vi "SUB_NI_Close_COM9.vi"() -> (0 "error":i32)   [LabVIEW 2011]
doc: "Closes the specified port."
panel:
  # "Problem: \nI want to make LabVIEW temporarily give up access to a serial port so that other programs can access it, \nbut I can't find a VI that will close my serial port. How can I do this?\n\nSolution: \nYou can use a lower level serial VI called Close Serial Driver.vi. \nIn LabVIEW 5.x, this VI is found under \\Labview\\vi.lib\\Instr\\_sersup.llb. In LabVIEW 6.0, \nit is located under \\LabVIEW 6\\vi.lib\\instr\\Serial.llb. If you include this VI in the application, \nit will allow other programs to use the serial port without having to exit LabVIEW. You can then re-access the port in LabVIEW by \nsubsequently running Serial Port Init.vi, and Serial Write.vi, or Serial Read.vi. \n\nOpening and closing serial ports in LabVIEW can also be done using VISA. This is done with VISA Open.vi and VISA Close.vi."
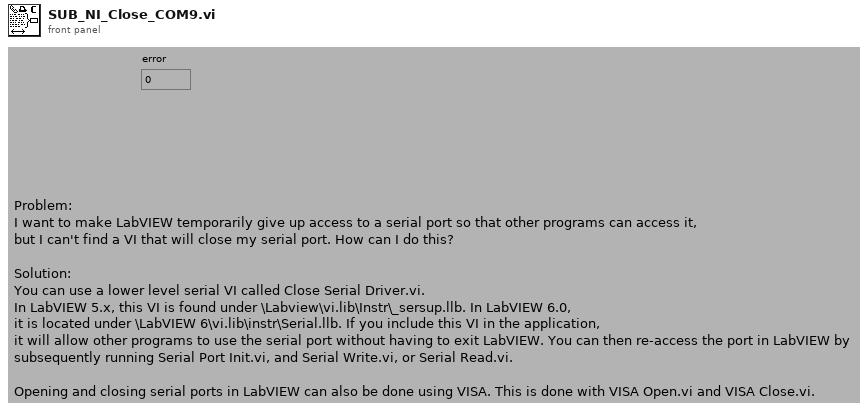
[diagram p1: front panel]
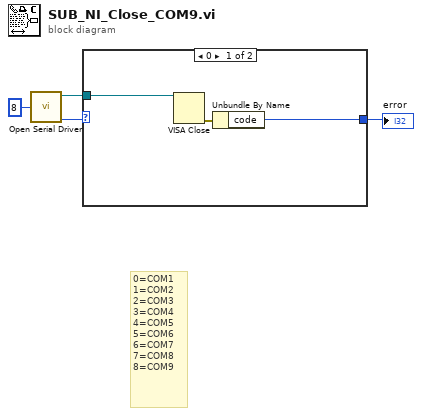
[diagram p0: block diagram]
diagram:
  # "0=COM1\n1=COM2\n2=COM3\n3=COM4\n4=COM5\n5=COM6\n6=COM7\n7=COM8\n8=COM9"
  n1 = call <vilib>:"Open Serial Driver.vi"("port number"=u32 8) -> ("input refnum"=w3:refnum<visa-resource-name>, "output error"=w4:i32)  [unwired: 2 out]
  n2 = case shown="0" w4 {
    selector: w4 -> [_ w8]
    tunnel: w3 -> [w7 _]
    tunnel: [w5 w8] -> w2
    frame 0 {
      n3 = VISA Close(VISA resource name=w7) -> (error out=w6:errorcluster)  [unwired: 1 in]
      n4 = Unbundle By Name(w6) -> ("code"=w5:i32)
    }
    frame 1, Default {
    }
  }
  "error" <- w2
